vi "Read NI-Scope Lock-in Configuration.vi"(8 "error in (no error)":errorcluster, 11 "NI-Scope Lock-in Driver in":refnum<class "NI-Scope Lock-in Driver.lvclass">) -> (0 "error out":errorcluster, 2 "Configuration":T1={"Pulse Configuration"={"Pre-trigger duration"=0.01, "Post-trigger duration"=0.1, "Rate"=1000000.0, "Ranges"=[10.0], "Re-name channels"=[], "Active channels"="0:1", "External clock"=FALSE}, "Points per sine wave"=0} {"Pulse Configuration"."Rate" format="%#_8pHz"; "Pulse Configuration"."Post-trigger duration" format="%#_6ps"; "Pulse Configuration"."Pre-trigger duration" format="%#_6ps"; "Pulse Configuration"."Ranges" format="%#_6pV"}, 3 "NI-Scope Lock-in Driver out":refnum<class "NI-Scope Lock-in Driver.lvclass">)   [LabVIEW 2016, in "NI-Scope Lock-in Driver.lvclass"]
uses:
  NI-Scope Lock-in Driver.lvclass
  C:/github/NHMFL_Core/Libraries/Instruments/Instrument Driver/Instrument Driver.lvclass
  NI-Scope Lock-in Configuration.ctl
  Instruments/Pulse Driver/Pusle Driver Configuration.ctl
  Instruments/Instrument Driver/Read User configuration.vi
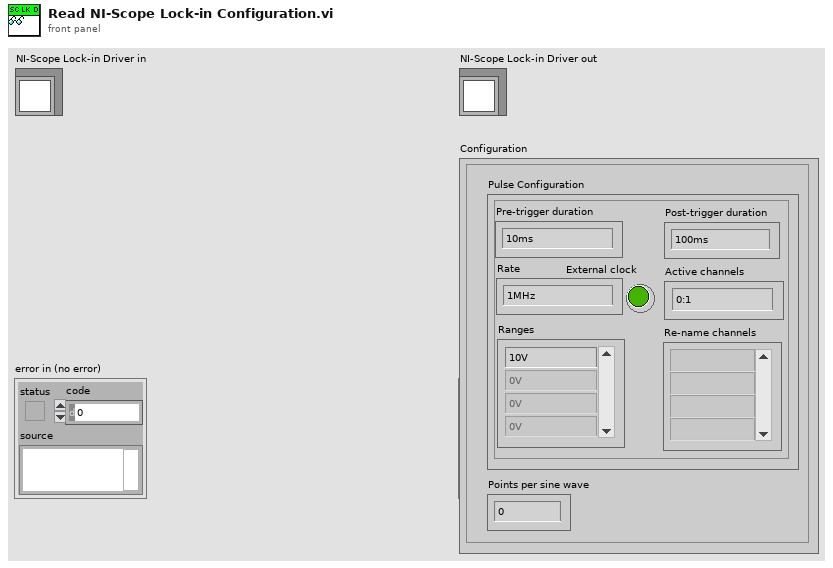
[diagram p1: front panel]
types:
  T1 = typedef "NI-Scope Lock-in Configuration.ctl" = cluster{"Pulse Configuration":T2, "Points per sine wave":i32}
  T2 = typedef "Pusle Driver Configuration.ctl" = cluster{"Pre-trigger duration":dbl, "Post-trigger duration":dbl, "Rate":dbl, "Ranges":dbl[], "Re-name channels":string[], "Active channels":string, "External clock":bool}
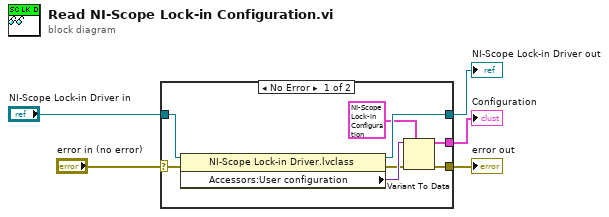
[diagram p0: block diagram]
diagram:
  n1 = case shown="No Error" "error in (no error)" {
    selector: "error in (no error)" -> [w13 w14]
    tunnel: [w6 w14] -> w4
    tunnel: [w11 w15] -> w2
    tunnel: "NI-Scope Lock-in Driver in" -> [w12 w15]
    tunnel: [w8 _] -> w1
    frame No Error {
      n2 = property class="NI-Scope Lock-in Driver.lvclass"(reference=w12, error in=w13) -> (reference out=w11:refnum<class "NI-Scope Lock-in Driver.lvclass">, error out=w7:errorcluster, "Accessors:User configuration"=w10:variant)
      n3 = Variant To Data(error in=w7, type=T1 {"Pulse Configuration"={"Pre-trigger duration"=0.01, "Post-trigger duration"=0.1, "Rate"=1000000.0, "Ranges"=[10.0], "Re-name channels"=[], "Active channels"="0:1", "External clock"=FALSE}, "Points per sine wave"=0} ("Configuration"), Variant=w10) -> (data=w8:T1, error out=w6:errorcluster)
    }
    frame Error {
    }
  }
  "error out" <- w4
  "NI-Scope Lock-in Driver out" <- w2
  "Configuration" <- w1
